vi "Error - Initialize.vi"(8 "error in (no error)":errorcluster, 11 "VI In":refnum<vi>) -> (0 "error out":errorcluster, 3 "Event Registration Out":refnum<event-registration>)   [LabVIEW 2024, in "Error Handler.lvlib"]
uses:
  Error Handler.lvlib
  Support/User Events/User Events.lvlib
  Error Queue - Create.vi
  Error Queue - Enqueue.vi
  Support/User Events/User Events - Register Events.vi
  Support/General Type Defs/User Events Cluster.ctl
  Support/General Type Defs/General Type Definitions.lvlib
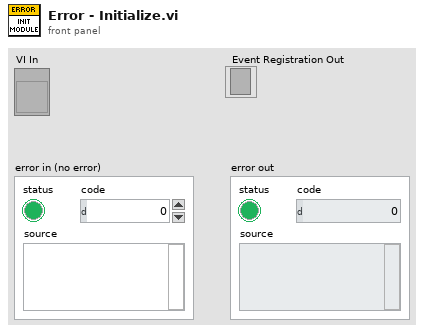
[diagram p1: front panel]
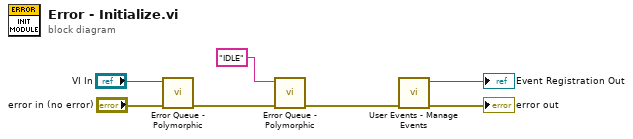
[diagram p0: block diagram]
diagram:
  n1 = call-poly "Error Queue - Polymorphic.vi"("error in"="error in (no error)", "VI In"="VI In") -> ("error out"=w3:errorcluster)  [unwired: 9 in]
  n2 = call-poly "Error Queue - Polymorphic.vi"("error in"=w3, "Message"="IDLE") -> ("error out"=w2:errorcluster)  [unwired: 9 in]
  n3 = call-poly "User Events - Manage Events.vi"("error in"=w2) -> ("error out"=→"error out":errorcluster, "Event Registration Out"=→"Event Registration Out":refnum<event-registration>)  [unwired: 9 in]
